vi "5 While loop.vi"() -> ()   [LabVIEW 2015]
panel:
  out "Iterations":i32
  in  "stop":bool
  out "EXCESSIVE":bool
  out "SAFE":bool
  out "Thermometer":dbl(slide) scale=0.0..100.0
  in  "Set Point":dbl
  in  "Temperature Sensor":dbl(knob) scale=0.0..100.0
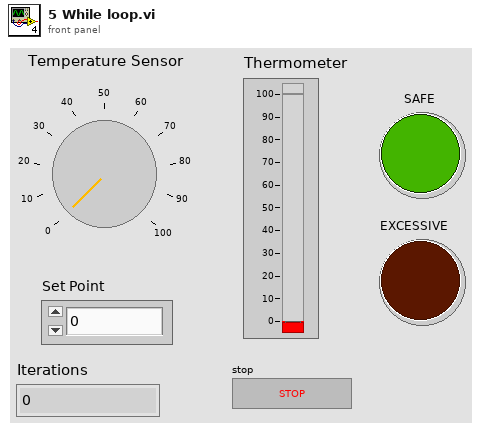
[diagram p1: front panel]
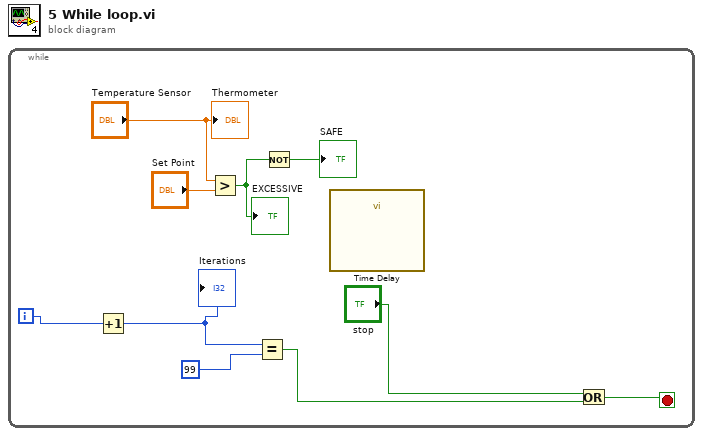
[diagram p0: block diagram]
diagram:
  n1 = while {
    i -> [w2]
    stop <- w6 stop-if-true
    n2 = Increment(x=w2) -> (x+1=w1:i32)
    "Iterations" <- w1
    n3 = Greater?(x="Temperature Sensor", y="Set Point") -> (0:w8:bool)
    "EXCESSIVE" <- w8
    n4 = Equal?(x=w1, y=99) -> (x = y?=w3:bool)
    n5 = Not(x=w8) -> (.not. x?=→"SAFE":bool)
    n6 = call "Time Delay"() -> ()  [unwired: 11 in, 1 out]
    n7 = Or(x="stop", y=w3) -> (x .or. y?=w6:bool)
    "Thermometer" <- "Temperature Sensor"
  }
